vi "DSF.Engine.Sequencer.Create.vi"(8 "error in (no error)":errorcluster, 10 "Plugin Runtimes":refnum<class "DSF.Engine.Plugin.Runtime.lvclass">[](array[class]), 11 "Sequencer type":refnum<class "DSF.Engine.Sequencer.lvclass">) -> (0 "error out":errorcluster, 3 "Sequencer":refnum<class "DSF.Engine.Sequencer.lvclass">)   [LabVIEW 2016, in "DSF.Engine.lvlib" / "DSF.Engine.Sequencer.lvclass"]
uses:
  DSF.Engine.Sequencer.lvclass
  DSF.Engine.Sequencer.Timing Bundle.lvclass
  Runtime/DSF.Engine.Runtime.lvclass
  Plugin/DSF.Engine.Plugin.Runtime.lvclass
  C:/Git/Sourcetree/DSF/Source/Engine/Classes/Runtime/DSF.Engine.Runtime.lvclass
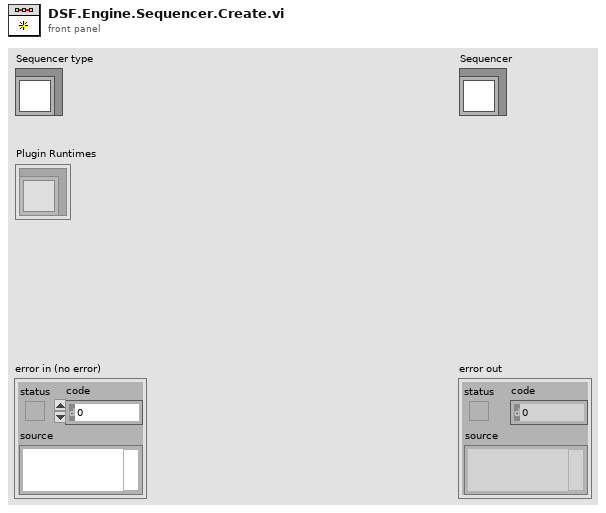
[diagram p1: front panel]
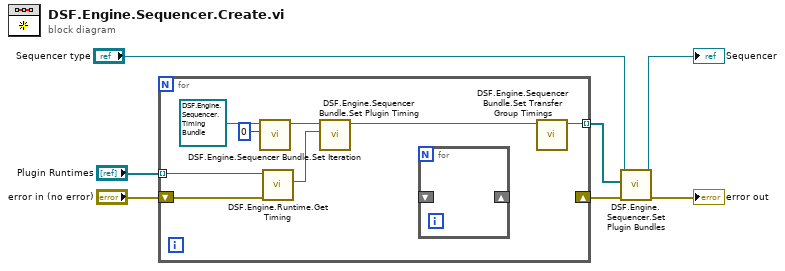
[diagram p0: block diagram]
diagram:
  n1 = for {
    tunnel: "Plugin Runtimes" -> [w15] mode=indexing
    shift-right: [_] -> w1
    shift-left: "error in (no error)" -> [w14]
    tunnel: [w9] -> w5 mode=indexing
    n2 = call "DSF.Engine.Sequencer Bundle.Set Iteration.vi"("iteration"=u64 0, "Sequencer Bundle in"=refnum<class "DSF.Engine.Sequencer.Timing Bundle.lvclass"> refnum ("DSF.Engine.lvlib:Sequencer Bundle.lvclass")) -> ("Sequencer Bundle out"=w12:refnum<class "DSF.Engine.Sequencer.Timing Bundle.lvclass">)  [unwired: 8 in, 1 out]
    n3 = call "DSF.Engine.Runtime.Get Timing.vi"("error in (no error)"=w14, "Runtime in"=w15) -> ("Timing"=w8:refnum<class "DSF.Shared.Timing.lvclass">)  [unwired: 7 in, 2 out]
    n4 = call "DSF.Engine.Sequencer Bundle.Set Plugin Timing.vi"("Plugin Timing"=w8, "Sequencer Bundle in"=w12) -> ("Sequencer Bundle out"=w10:refnum<class "DSF.Engine.Sequencer.Timing Bundle.lvclass">)  [unwired: 8 in, 1 out]
    n5 = for {
      shift-right: _ -> [_]
      shift-left: _ -> [_]
    }
    n6 = call "DSF.Engine.Sequencer Bundle.Set Transfer Group Timings.vi"("Sequencer Bundle in"=w10) -> ("Sequencer Bundle out"=w9:refnum<class "DSF.Engine.Sequencer.Timing Bundle.lvclass">)  [unwired: 9 in, 1 out]
  }
  n7 = call "DSF.Engine.Sequencer.Set Plugin Bundles.vi"("error in (no error)"=w1, "Plugin Bundles"=w5, "Sequencer in"="Sequencer type") -> ("error out"=→"error out":errorcluster, "Sequencer out"=→"Sequencer":refnum<class "DSF.Engine.Sequencer.lvclass">)  [unwired: 7 in]
